vi "Launched Nested Actors.vi"(8 "error in (no error)":errorcluster, 11 "Car Wash Controller in":refnum<class "Car Wash Controller.lvclass">) -> (0 "error out":errorcluster, 3 "Car Wash Controller out":refnum<class "Car Wash Controller.lvclass">)   [LabVIEW 2019, in "Car Wash Controller.lvlib" / "Car Wash Controller.lvclass"]
uses:
  Car Wash Controller.lvclass
  C:/Program Files (x86)/National Instruments/LabVIEW 2019/vi.lib/ActorFramework/Actor/Actor.lvclass
  Sim Entry Console Actor/Car Wash Controller/Sim Entry Console Actor.lvclass
  Sim Wash Display Console/Car Wash Controller/Sim Wash Display Console.lvclass
  Vehicle Position Simulation Actor/Car Wash Controller/Vehicle Position Simulation Actor.lvclass
  Sim Configuration Database Actor/Sim Configuration Database Actor/Sim Configuration Database Actor.lvclass
  Car Wash Controller.lvclass/Car Wash Controller.ctl
  <vilib>/ActorFramework/Actor/Actor.lvclass
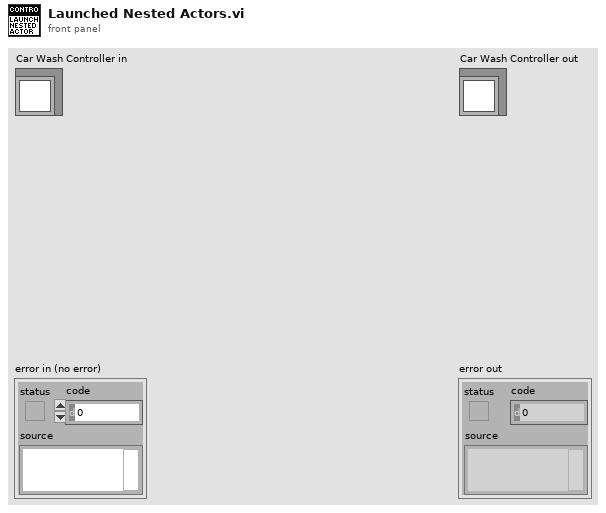
[diagram p1: front panel]
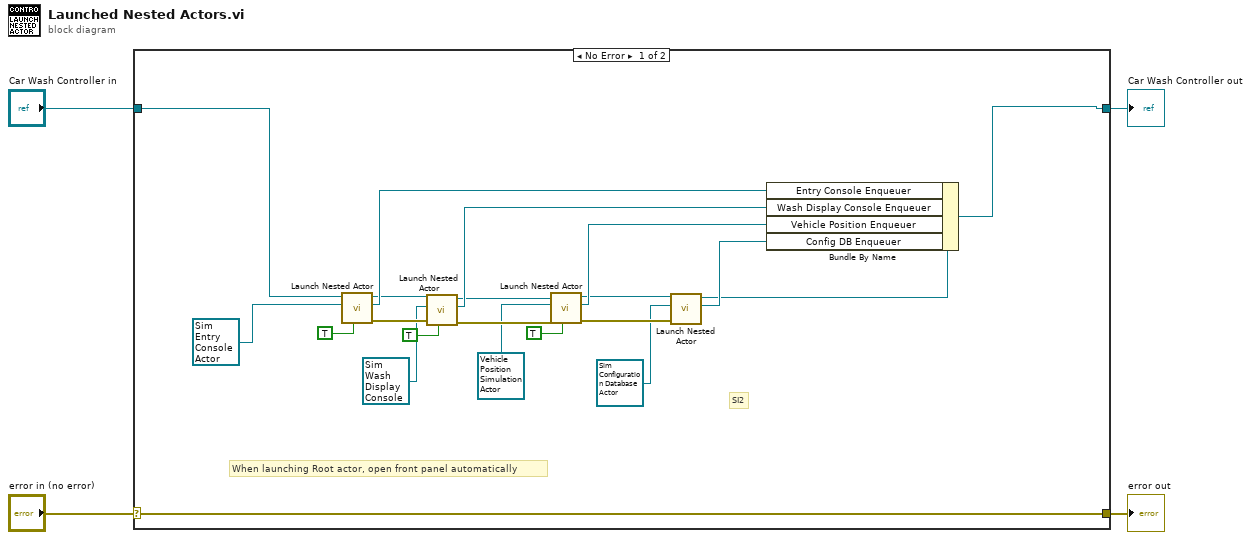
[diagram p0: block diagram]
diagram:
  n1 = case shown="No Error" "error in (no error)" {
    selector: "error in (no error)" -> [w25 w27]
    tunnel: [w25 w27] -> w3
    tunnel: [w21 w26] -> w1
    tunnel: "Car Wash Controller in" -> [w22 w26]
    frame No Error {
      # "SI2"
      # "When launching Root actor, open front panel automatically"
      n2 = call <vilib>:"Launch Nested Actor.vi"("Open Actor Core front panel? (F)"=TRUE, "Nested Actor"=refnum<class "Sim Entry Console Actor.lvclass"> refnum ("Sim Entry Console Actor.lvlib:Sim Entry Console Actor.lvclass"), "Caller Actor in"=w22) -> ("error out"=w18:errorcluster, "Nested Actor's Enqueuer"=w20:refnum<class "Message Enqueuer.lvclass">, "Caller Actor out"=w19:refnum<class "Car Wash Controller.lvclass">)  [unwired: 6 in]
      n3 = call <vilib>:"Launch Nested Actor.vi"("Open Actor Core front panel? (F)"=TRUE, "error in (no error)"=w18, "Nested Actor"=refnum<class "Sim Wash Display Console.lvclass"> refnum ("Sim Wash Display Console.lvlib:Sim Wash Display Console.lvclass"), "Caller Actor in"=w19) -> ("error out"=w13:errorcluster, "Nested Actor's Enqueuer"=w16:refnum<class "Message Enqueuer.lvclass">, "Caller Actor out"=w14:refnum<class "Car Wash Controller.lvclass">)  [unwired: 5 in]
      n4 = call <vilib>:"Launch Nested Actor.vi"("Open Actor Core front panel? (F)"=TRUE, "error in (no error)"=w13, "Nested Actor"=refnum<class "Vehicle Position Simulation Actor.lvclass"> refnum ("Vehicle Position Sinmulation Actor.lvlib:Vehicle Position Simulation Actor.lvclass"), "Caller Actor in"=w14) -> ("error out"=w8:errorcluster, "Nested Actor's Enqueuer"=w12:refnum<class "Message Enqueuer.lvclass">, "Caller Actor out"=w9:refnum<class "Car Wash Controller.lvclass">)  [unwired: 5 in]
      n5 = call <vilib>:"Launch Nested Actor.vi"("error in (no error)"=w8, "Nested Actor"=refnum<class "Sim Configuration Database Actor.lvclass"> refnum ("Sim Configuration Database Actor.lvlib:Sim Configuration Database Actor.lvclass"), "Caller Actor in"=w9) -> ("Nested Actor's Enqueuer"=w6:refnum<class "Message Enqueuer.lvclass">, "Caller Actor out"=w5:refnum<class "Car Wash Controller.lvclass">)  [unwired: 6 in, 1 out]
      n6 = Bundle By Name(cluster=w5, "Entry Console Enqueuer"=w20, "Wash Display Console Enqueuer"=w16, "Vehicle Position Enqueuer"=w12, "Config DB Enqueuer"=w6) -> (w21:refnum<class "Car Wash Controller.lvclass">)
    }
    frame Error {
    }
  }
  "error out" <- w3
  "Car Wash Controller out" <- w1
